vi "获取当天时间段.vi"(8 "24制小时数下限":i32, 9 "设置初始时间":string, 11 "24制小时数上限":i32=24) -> (0 "判断当前时间是否在规定时间内":bool, 1 "初始时间":string, 2 "当前时间":string, 3 "两位数时间":string)   [LabVIEW 2014]
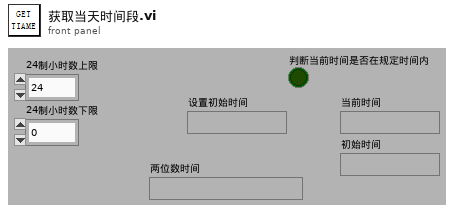
[diagram p1: front panel]
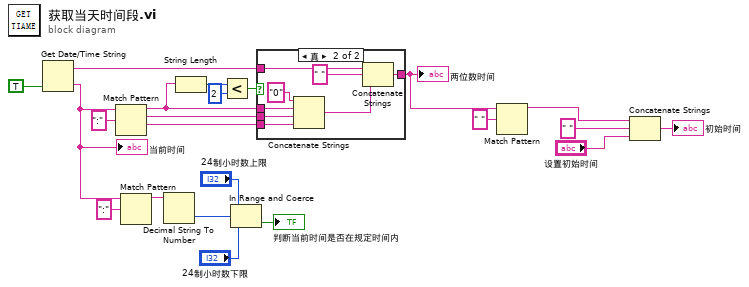
[diagram p0: block diagram]
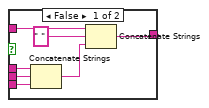
[diagram p2: hidden frame]
diagram:
  n1 = Get Date/Time String(want seconds? (F)=TRUE ("需要秒？(F)")) -> (date string=w20:string, time string=w4:string)  [unwired: 2 in]
  "当前时间" <- w4
  n2 = Match Pattern(string=w4, regular expression=":" ("正则表达式")) -> (before substring=w19:string, match substring=w21:string, after substring=w22:string)  [unwired: 1 in, 1 out]
  n3 = Match Pattern(string=w4, regular expression=":" ("正则表达式")) -> (before substring=w5:string)  [unwired: 1 in, 3 out]
  n4 = Decimal String To Number(string=w5) -> (number=w6:i32)  [unwired: 2 in, 1 out]
  n5 = String Length(string=w19) -> (length=w16:i32)
  n6 = Less?(x=w16, y=2) -> (x < y?=w18:bool)
  n7 = In Range and Coerce(upper limit="24制小时数上限", x=w6, lower limit="24制小时数下限") -> (In Range?=→"判断当前时间是否在规定时间内":bool)  [unwired: 1 out]
  n8 = case shown="真" w18 {
    tunnel: w19 -> [w27 w34]
    tunnel: w20 -> [w26 w37]
    tunnel: w21 -> [w24 w33]
    tunnel: w22 -> [w23 w32]
    tunnel: [w25 w30] -> w10
    frame False {
      n9 = Concatenate Strings(w27, w24, w23) -> (w28:string)
      n10 = Concatenate Strings(w26, " " ("字符串"), w28) -> (w25:string)
    }
    frame True {
      n11 = Concatenate Strings("0" ("字符串"), w34, w33, w32) -> (w31:string)
      n12 = Concatenate Strings(w37, " " ("字符串"), w31) -> (w30:string)
    }
  }
  "两位数时间" <- w10
  n13 = Match Pattern(string=w10, regular expression=" " ("字符串")) -> (before substring=w13:string)  [unwired: 1 in, 3 out]
  n14 = Concatenate Strings(w13, " " ("字符串"), "设置初始时间") -> (→"初始时间":string)
